vi "Fit phase one.vi"(8 "Error In":errorcluster, 9 "Initial parameters":dbl[](array[numeric])=[188.484, 0.01, 2.4] format="%#_6p", 10 "Z":cdb[](array[numeric]), 11 "X":dbl[](array[numeric])) -> (0 "Error Out":errorcluster, 1 "best fit parameters":dbl[](array[numeric]))   [LabVIEW 2016]
uses:
  <vilib>/gmath/NumericalOptimization/Nonlinear Curve Fit LM bound.vi
  <vilib>/gmath/NI_Gmath.lvlib
  <vilib>/Analysis/NI_AALPro.lvlib
panel:
  out "sqrt(x)":dbl
  out "Circle phase":dbl
  out "Circle plot":cluster{dbl[], dbl[]}[](graph)
  out "Phase in":cluster{"X":dbl[], dbl[]}(graph)
  out "Amplitude in":cluster{"X":dbl[], dbl[]}(graph)
  in  "Bounds":T1={"parameter minimum"=[1.0, 1.0, -6.3], "parameter maximum"=[10000000.0, 200.0, 10.0]} {"parameter minimum" format="%#_6p"}
  out "Weight":dbl[](graph)
  out "number of function calls":i32
  in  "termination":cluster{"max iteration":i32, "tolerance":dbl}={"max iteration"=200, "tolerance"=1e-08}
  out "Fit":cluster{"X":dbl[], "best nonlinear fit":dbl[]}[](graph)
  # "F0\nG\nA\nP\nX\nY"
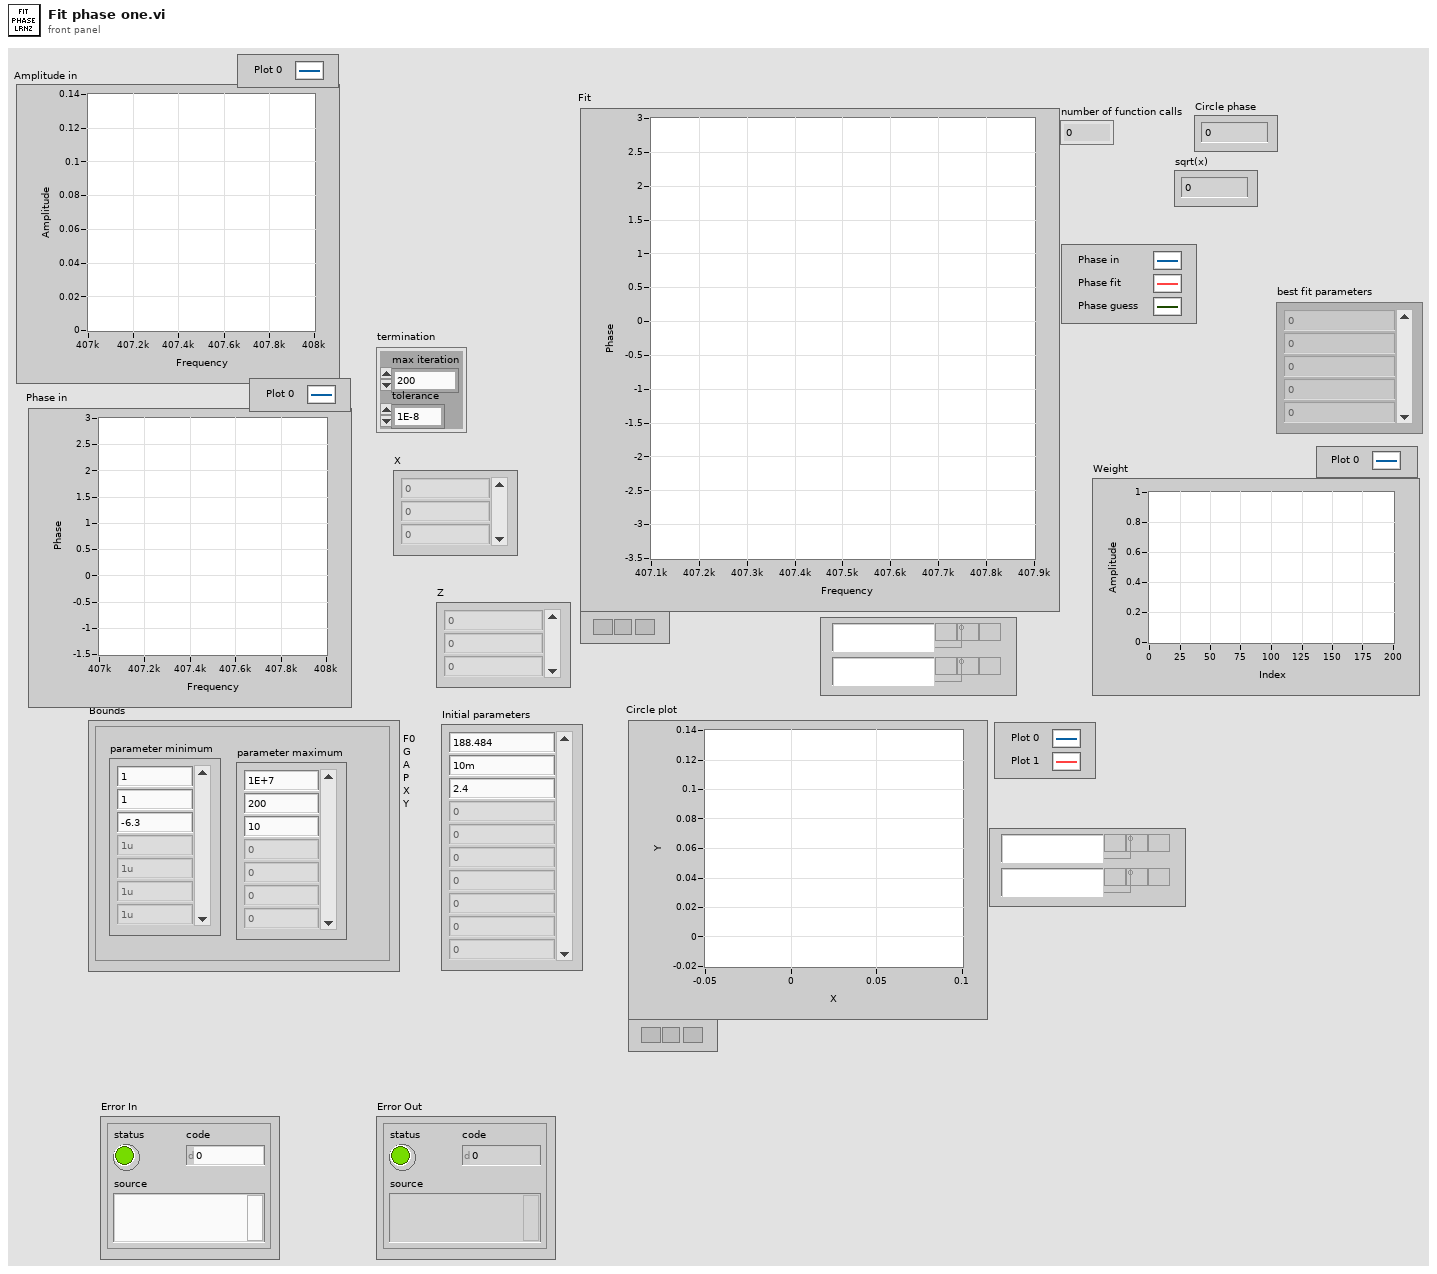
[diagram p1: front panel]
types:
  T1 = cluster{"parameter minimum":dbl[], "parameter maximum":dbl[]}
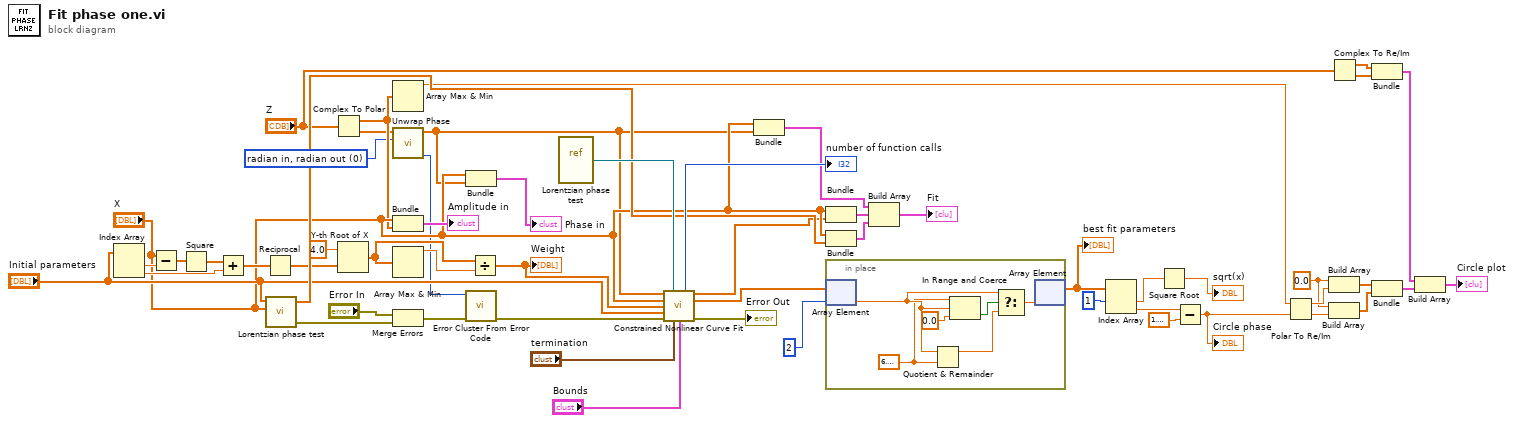
[diagram p0: block diagram]
diagram:
  w17 = 0 items=["radian in, radian out", "radian in, degree out", "degree in, degree out", "degree in, radian out"] ("phase unit")
  w28 = 0.0 ("element")
  n1 = Index Array(array="Initial parameters") -> (element #1=w46:dbl, element #2=w43:dbl)  [unwired: 2 in]
  n2 = Subtract(x="X", y=w46) -> (x-y=w45:dbl[])
  n3 = Square(x=w45) -> (x^2=w44:dbl[])
  n4 = Add(x=w44, y=w43) -> (x+y=w42:dbl[])
  n5 = Reciprocal(x=w42) -> (1/x=w12:dbl[])
  n6 = call "Lorentzian phase test.vi"("X"="X", "a"="Initial parameters") -> ("error out"=w3:errorcluster, "f(X,a)"=w48:dbl[])  [unwired: 2 in, 1 out]
  n7 = Complex To Polar(r * e^(i*theta)="Z") -> (r=w31:dbl[], theta=w16:dbl[])
  n8 = Y-th Root of X(1:w12, 2:4.0) -> (0:w10:dbl[])
  n9 = Array Max & Min(array=w31) -> (max value=w30:dbl)  [unwired: 3 out]
  n10 = call <vilib>:"Unwrap Phase.vi"("phase unit"=w17, "Phase"=w16) -> ("error"=w6:i32, "Unwrapped Phase"=w15:dbl[])  [unwired: 8 in]
  n11 = Bundle("X"="X", w31) -> (→"Amplitude in":cluster{"X":dbl[], dbl[]})  [unwired: 1 in]
  n12 = Array Max & Min(array=w10) -> (max value=w41:dbl)  [unwired: 3 out]
  n13 = Merge Errors("Error In", w3) -> (w4:errorcluster)
  n14 = Bundle("X"="X", "Unwrapped Phase"=w15) -> (→"Phase in":cluster{"X":dbl[], "Unwrapped Phase":dbl[]})  [unwired: 1 in]
  n15 = call <vilib>:"Error Cluster From Error Code.vi"("error in (no error)"=w4, "error code (0)"=w6) -> ("error out"=w2:errorcluster)  [unwired: 7 in]
  n16 = Divide(x=w10, y=w41) -> (x/y=w14:dbl[])
  "Weight" <- w14
  n17 = vi-ref "Lorentzian phase test.vi"() -> (w55:refnum<vi>)
  n18 = call-poly <vilib>:"Constrained Nonlinear Curve Fit.vi"("Y"=w15, "f(x,a)"=w55, "X"="X", "Weight"=w14, "initial parameters"="Initial parameters", "error in (no error)"=w2, "termination"="termination", "parameter bounds"="Bounds") -> ("number of function calls"=→"number of function calls":i32, "best nonlinear fit"=w36:dbl[], "best fit parameters"=w9:dbl[], "error out"=→"Error Out":errorcluster)  [unwired: 2 in, 2 out]
  n19 = Bundle("X"="X", "Unwrapped Phase"=w15) -> (w50:cluster{"X":dbl[], "Unwrapped Phase":dbl[]})  [unwired: 1 in]
  n20 = Bundle("X"="X", "best nonlinear fit"=w36) -> (w49:cluster{"X":dbl[], "best nonlinear fit":dbl[]})  [unwired: 1 in]
  n21 = Bundle("X"="X", "f(X,a)"=w48) -> (w51:cluster{"X":dbl[], "f(X,a)":dbl[]})  [unwired: 1 in]
  n22 = in-place {
    w58 = 6.283185307179586
    n23 = in-place-array #1(w9, 2) -> (w59:dbl)
    n24 = Quotient & Remainder(x=w59, y=w58) -> (x-y*floor(x/y)=w57:dbl)  [unwired: 1 out]
    n25 = In Range and Coerce(upper limit=w58, x=w59, lower limit=0.0) -> (In Range?=w60:bool)  [unwired: 1 out]
    n26 = Select(t=w59, s=w60, f=w57) -> (s? t:f=w56:dbl)
    n27 = in-place-array #1(w56) -> (w8:dbl[])  [unwired: 1 out]
  }
  "best fit parameters" <- w8
  n28 = Build Array(w50, w49, w51) -> (→"Fit":cluster{"X":dbl[], "f(X,a)":dbl[]}[])
  n29 = Index Array(array=w8, index #1=1 ("index")) -> (element #1=w19:dbl, element #2=w20:dbl)  [unwired: 1 in]
  n30 = Square Root(x=w19) -> (sqrt(x)=→"sqrt(x)":dbl)
  n31 = Subtract(x=w20, y=1.5707963267948966) -> (x-y=w13:dbl)
  "Circle phase" <- w13
  n32 = Polar To Re/Im(2:w13, 3:w30) -> (0:w27:dbl, 1:w29:dbl)
  n33 = Build Array(w28, w29) -> (w26:dbl[])
  n34 = Build Array(w28, w27) -> (w25:dbl[])
  n35 = Complex To Re/Im(x + iy="Z") -> (x=w34:dbl[], y=w33:dbl[])
  n36 = Bundle(w34, w33) -> (w32:cluster{dbl[], dbl[]})  [unwired: 1 in]
  n37 = Bundle(w26, w25) -> (w23:cluster{dbl[], dbl[]})  [unwired: 1 in]
  n38 = Build Array(w32, w23) -> (→"Circle plot":cluster{dbl[], dbl[]}[])
